vi "set_enabled_status.vi"(8 "error in (no error)":errorcluster, 10 "enabled?":bool, 11 "ClockDL090202FPGA in":refnum<class "ClockDL090202FPGA.lvclass">) -> (0 "error out":errorcluster, 3 "ClockDL090202FPGA out":refnum<class "ClockDL090202FPGA.lvclass">)   [LabVIEW 2010, in "ClockDL090202FPGA.lvclass"]
uses:
  ClockDL090202FPGA.lvclass
  GenericClock/GenericClock/GenericClock.lvclass
  ClockDL090202FPGA.lvclass/ClockDL090202FPGA.ctl
  FPGAWrapper/GenericFPGAWrapper/GenericFPGAWrapper/GenericFPGAWrapper.lvclass
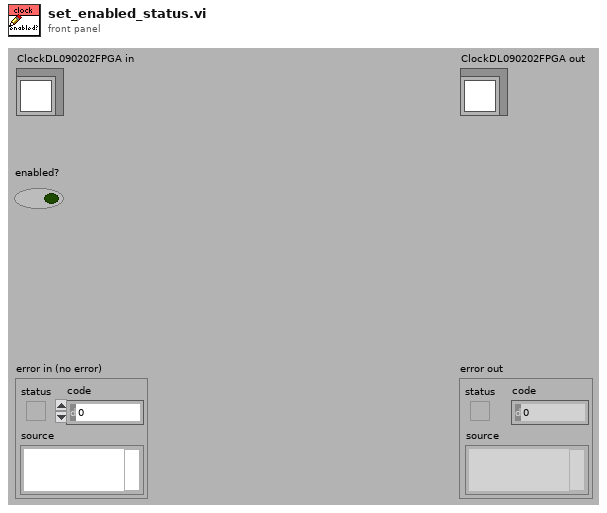
[diagram p1: front panel]
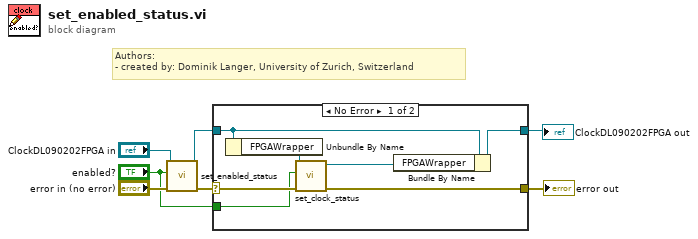
[diagram p0: block diagram]
diagram:
  # "Authors: \n- created by: Dominik Langer, University of Zurich, Switzerland"
  n1 = call-parent "set_enabled_status.vi"("error in (no error)"="error in (no error)", "enabled?"="enabled?", "GenericClock in"="ClockDL090202FPGA in") -> ("error out"=w5:errorcluster, "GenericClock out"=w4:refnum<class "ClockDL090202FPGA.lvclass">)  [unwired: 7 in]
  n2 = case shown="No Error" w5 {
    selector: w5 -> [w13 w16]
    tunnel: w4 -> [w9 w15]
    tunnel: [w12 w16] -> w3
    tunnel: [w8 w15] -> w2
    tunnel: "enabled?" -> [w11 _]
    frame No Error {
      n3 = Unbundle By Name(w9) -> ("FPGAWrapper"=w14:refnum<class "GenericFPGAWrapper.lvclass">)
      n4 = call-dynamic "set_clock_status.vi"("error in (no error)"=w13, "enable clocks?"=w11, "GenericFPGAWrapper in"=w14) -> ("error out"=w12:errorcluster, "GenericFPGAWrapper out"=w10:refnum<class "GenericFPGAWrapper.lvclass">)  [unwired: 7 in]
      n5 = Bundle By Name(cluster=w9, "FPGAWrapper"=w10) -> (w8:refnum<class "ClockDL090202FPGA.lvclass">)
    }
    frame Error {
    }
  }
  "error out" <- w3
  "ClockDL090202FPGA out" <- w2
